vi "read metadata property.vi"(8 "error in":errorcluster, 10 "key":string, 11 "configuration in":refnum<class "TBM configuration.lvclass">) -> (0 "error out":errorcluster, 1 "value":string, 2 "found":bool, 3 "configuration out":refnum<class "TBM configuration.lvclass">)   [LabVIEW 2013, in "TBM configuration.lvclass"]
doc: "Reads a single string property from the set of key/value pairs stored in the configuration class."
uses:
  TBM configuration.lvclass
  TBM configuration.lvclass/TBM configuration.ctl
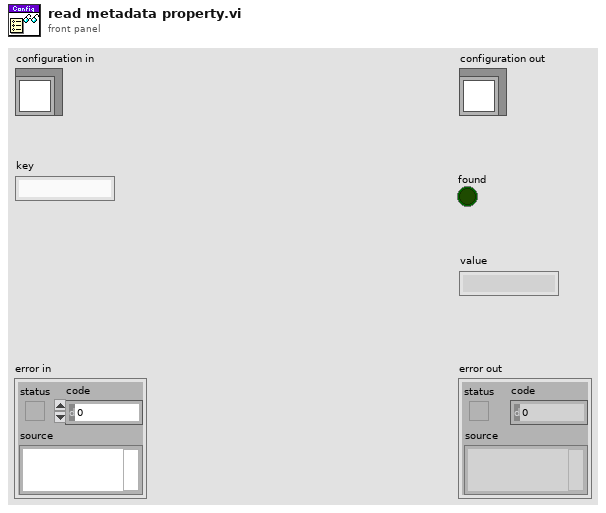
[diagram p1: front panel]
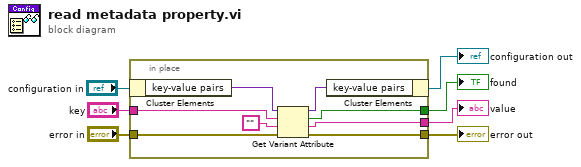
[diagram p0: block diagram]
diagram:
  n1 = in-place {
    in-place-border: "key" -> [w12]
    in-place-border: "error in" -> [w11]
    in-place-border: [w10] -> w3
    in-place-border: [w9] -> w2
    in-place-border: [w8] -> w1
    n2 = in-place-cluster #1("configuration in") -> ("key-value pairs"=w15:variant)
    n3 = Get Variant Attribute(Variant=w15, name=w12, default value (empty Variant)="", error in=w11) -> (duplicate Variant=w14:variant, found=w8:bool, value=w9:string, error out=w10:errorcluster)
    n4 = in-place-cluster #1("key-value pairs"=w14) -> (→"configuration out":refnum<class "TBM configuration.lvclass">)
  }
  "error out" <- w3
  "value" <- w2
  "found" <- w1
